vi "motioncontrol.vi"() -> ()   [LabVIEW 2016]
uses:
  GitHub/UCSB-Gantry/V5/Drivers/Aerotech A3200/Motion/MoveAbsSingle.vi
  GitHub/UCSB-Gantry/V5/Drivers/Aerotech A3200/Aerotech VIs.lvlib
panel:
  in  "Radius":dbl
  in  "Y Endpoint":dbl
  in  "X Endpoint":dbl
  in  "Make Circle":bool
  out "Z Position":dbl
  out "X Position":dbl
  out "Theta Position":dbl
  out "Y Position":dbl
  in  "Joystick ON/OFF":bool
  in  "Incrimental":bool
  in  "Angular position":dbl
  in  "Angular rotation":dbl
  in  "Theta-Go":bool
  in  "Abs distance":dbl
  in  "Incrimental":bool
  in  "Inc distance":dbl
  in  "Z-Go":bool
  in  "Square Speeds":dbl[](array[numeric])=[0.0, 0.0, 0.0]
  in  "Square Sizes":dbl[](array[numeric])=[0.0, 0.0, 0.0]
  in  "XY Go":bool
  in  "Make CW square":bool
  in  "positions/abs":dbl[](array[numeric])=[0.0, 0.0]
  in  "distances/linear":dbl[](array[numeric])=[0.0, 0.0]
  in  "Linear":bool
  in  "STOP PROGRAM":bool
  # "XY Motion"
  # "Theta"
  # "X"
  # "Y"
  # "Absolute"
  # "abs"
  # "Z-Control"
  # "Shapes"
  # "Absolute"
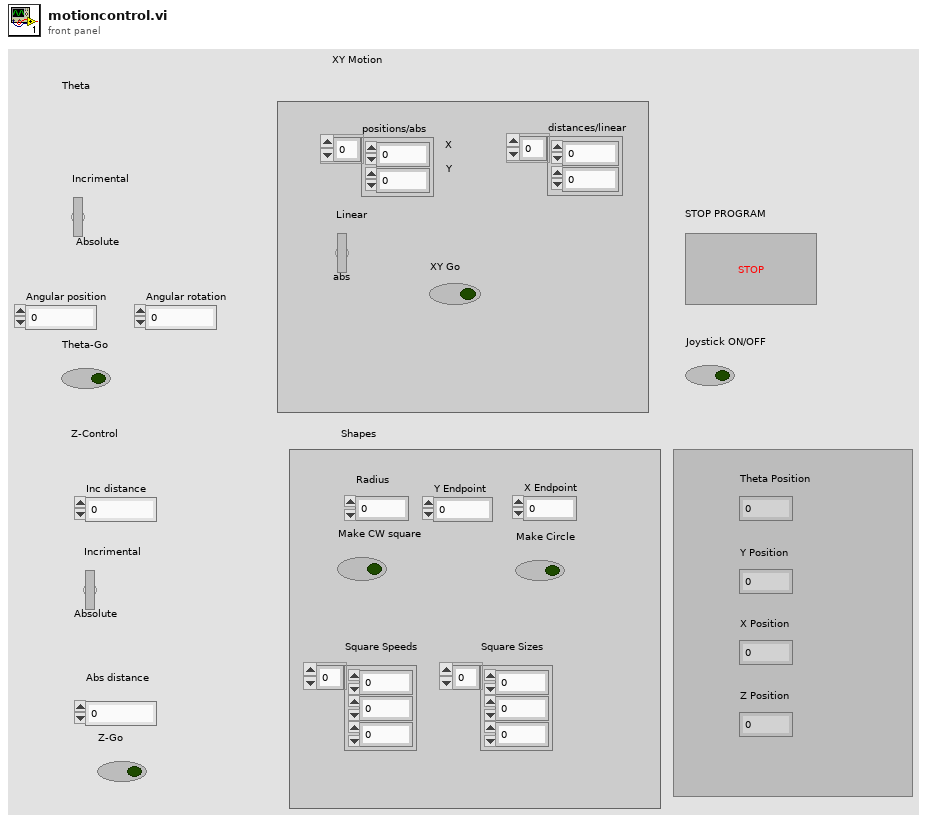
[diagram p1: front panel]
types:
  T1 = typedef "Aerotech VIs.lvlib/ControllerDiagPacket.ctl" = cluster{"Number of Diag Packets":i32, "Axes":T2[], "error":errorcluster}
  T2 = typedef "Aerotech VIs.lvlib/AxisDiagPacket.ctl" = cluster{"Axis Name":string, "Analog Input 0":dbl, "Analog Input 1":dbl, "Axis Fault (num)":i32, "Axis Fault (str)":string, "Axis Fault (bits)":cluster{"AmplifierFault":bool, "AmplifierTemperatureFault":bool, "CcwEndOfTravelLimitFault":bool, "CcwSoftwareLimitFault":bool, "CommunicationLostFault":bool, "CwEndOfTravelLimitFault":bool, "CwSoftwareLimitFault":bool, "EmergencyStopFault":bool, "EncoderFault":bool, "ExternalFault":bool, "FeedbackScalingFault":bool, "GantryMisalignFault ":bool, "HallSensorFault":bool, "InPositionTimeoutFault":bool, "MarkerSearchFault":bool, "MaxVelocityCommandFault":bool, "MotorTemperatureFault":bool, "None":bool, "OverCurrentFault":bool, "PositionErrorFault":bool, "PositionFeedbackFault":bool, "PowerSupplyFault":bool, "ProbeInputFault":bool, "SafeZoneFault":bool, "VelocityErrorFault":bool, "VelocityFeedbackFault":bool, "VoltageClampFault":bool}, "Axis Status (num)":i32, "Axis Status (str)":string, "Axis Status (bits)":cluster{"BacklashActive":bool, "CalibrationEnabled1D":bool, "CalibrationEnabled2D":bool, "CommandValid":bool, "DriveAbortPending":bool, "DrivePending":bool, "Enabling":bool, "GainMappingEnabled":bool, "GantryAligned":bool, "GantryRealigning":bool, "Homed":bool, "Homing":bool, "IFOVEnabled":bool, "JogGenerating":bool, "Jogging":bool, "JoystickControl":bool, "MasterSlaveControl":bool, "MotionBlocked":bool, "MotionClamped":bool, "MoveDone":bool, "None":bool, "NotVirtual":bool, "Profiling":bool, "Stability0":bool, "Stability1":bool, "TrajectoryFiltering":bool, "WaitDone":bool}, "Current Command":sgl, "Current Error":sgl, "Current Feedback":sgl, "Digital Inputs":i32, "Digital Outputs":i32, "Drive Status":i32, "Drive Status (str)":string, "Drive Status (bits)":cluster{"AccelerationPhase":bool, "AutofocusActive":bool, "BrakeOutput":bool, "CcwEndOfTravelLimitInput":bool, "CosineEncoderError":bool, "CurrentClamp":bool, "CwEndOfTravelLimitInput":bool, "DecelerationPhase":bool, "DualLoopActive":bool, "EmergencyStopInput":bool, "Enabled":bool, "EncoderClipping":bool, "GalvoCalibrationEnabled":bool, "GalvoPowerCorrection":bool, "HallAInput":bool, "HallBInput":bool, "HallCInput":bool, "HighResolutionMode":bool, "HomeLimitInput":bool, "InPosition":bool, "InPosition2":bool, "MarkerInput":bool, "MarkerLatch":bool, "MoveActive":bool, "NoMotorSupply":bool, "None":bool, "PowerLimiting":bool, "ProgrammingFlash":bool, "ProgrammingMXH":bool, "PSOHaltLatch":bool, "ServoControl":bool, "SineEncoderError":bool}, "Position Feedback Auxiliary":dbl, "Position Command":dbl, "Position Error":dbl, "Position Feedback":dbl, "Program Position Command":dbl, "Program Position Error":dbl, "Program Position Feedback":dbl, "Velocity Command":dbl, "Velocity Error":dbl, "Velocity Feedback":dbl}
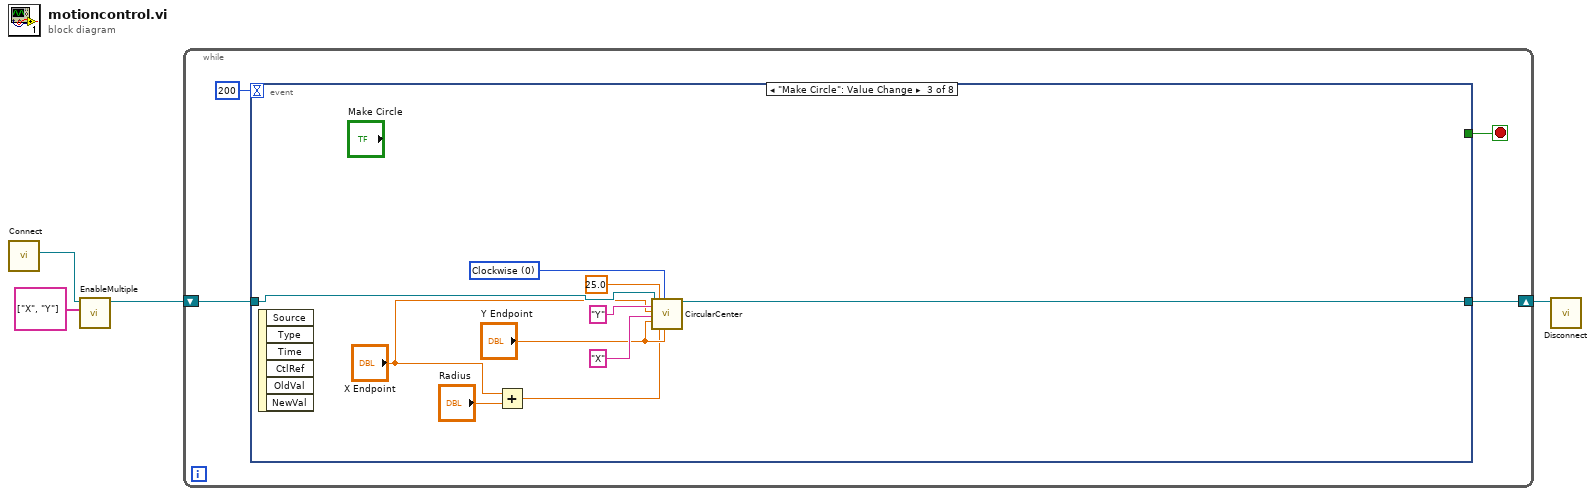
[diagram p0: block diagram]
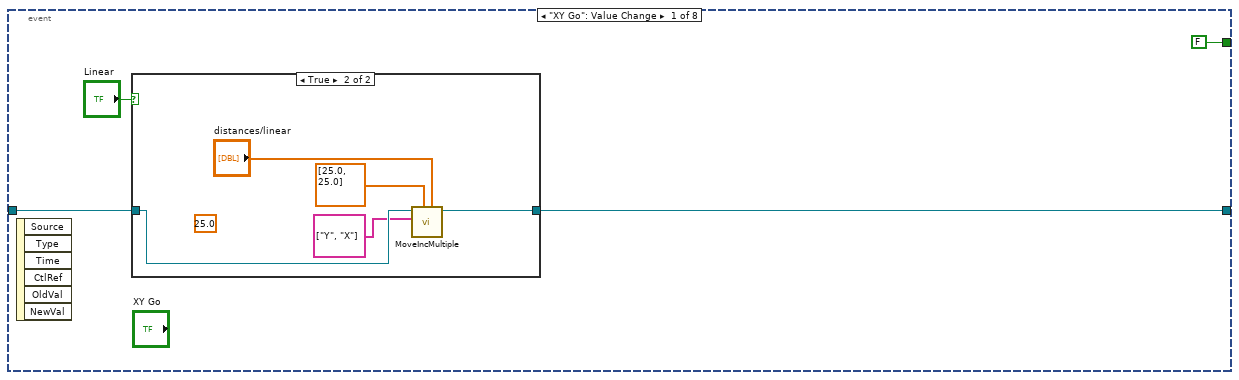
[diagram p2: hidden frame]
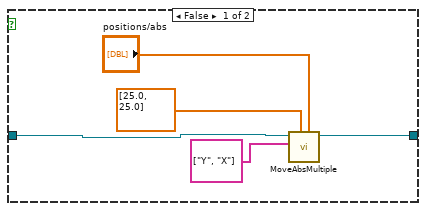
[diagram p3: hidden frame]
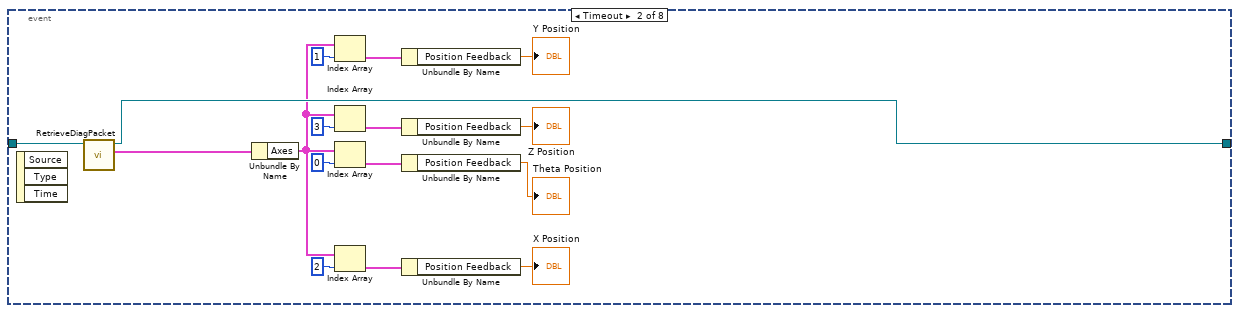
[diagram p4: hidden frame]
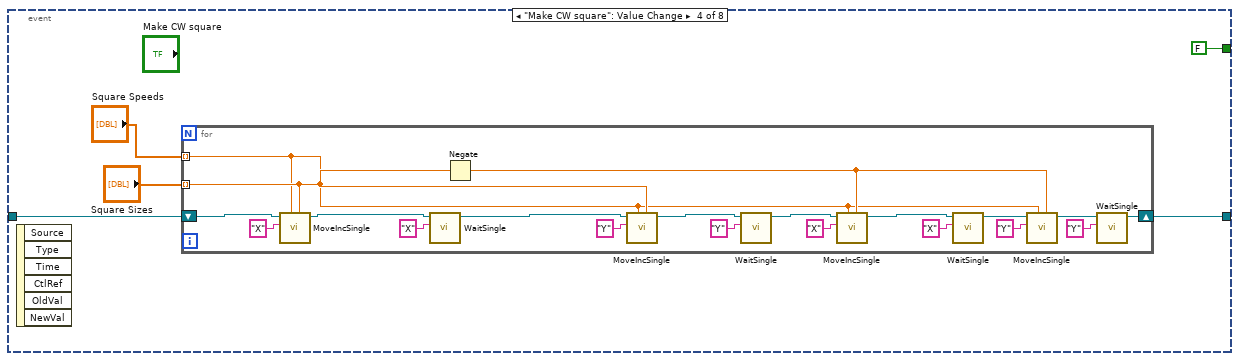
[diagram p5: hidden frame]
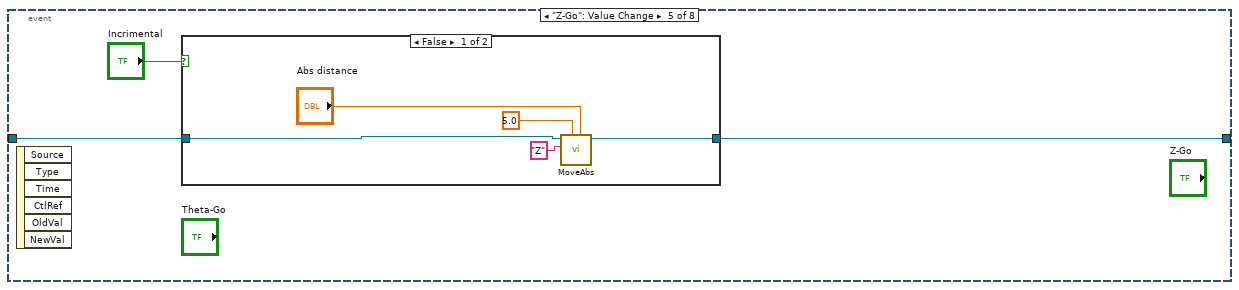
[diagram p6: hidden frame]
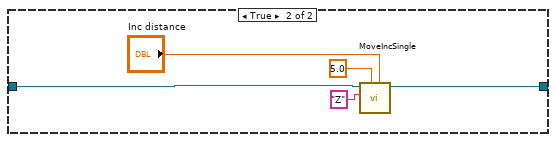
[diagram p7: hidden frame]
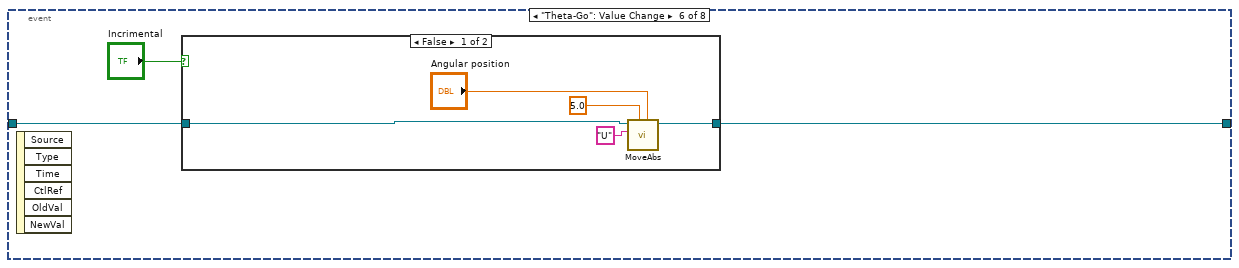
[diagram p8: hidden frame]
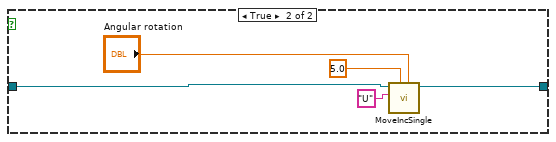
[diagram p9: hidden frame]
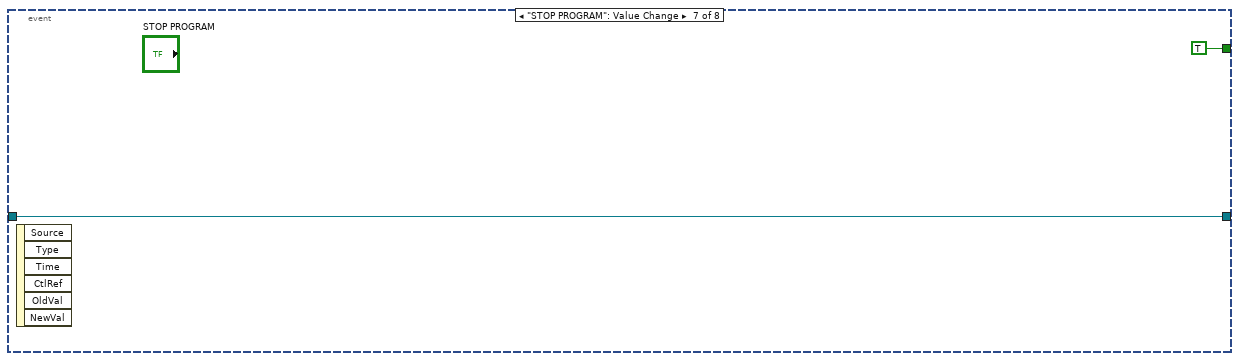
[diagram p10: hidden frame]
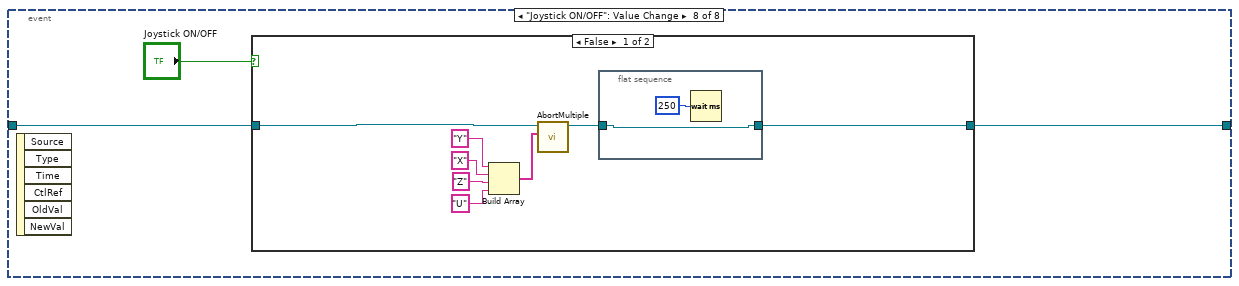
[diagram p11: hidden frame]
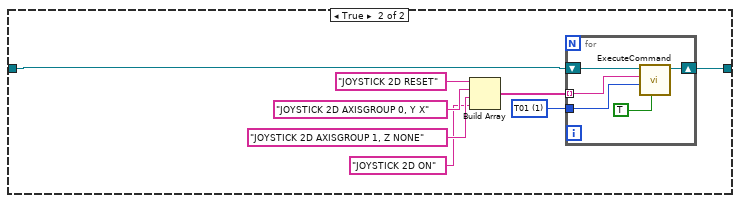
[diagram p12: hidden frame]
diagram:
  n1 = call "Connect.vi"() -> ("controller"=w4:refnum<k24>)  [unwired: 10 in, 1 out]
  n2 = call "EnableMultiple.vi"("axis names"=string[] ["X", "Y"], "controller in"=w4) -> ("controller out"=w2:refnum<k24>)  [unwired: 8 in, 1 out]
  n3 = while {
    shift-right: [w6] -> w1
    shift-left: w2 -> [w8]
    stop <- w7 stop-if-true
    n4 = event shown="[2] \"Make Circle\": Value Change" {
      selector: _ -> [_ _ _ _ _ _ _ _]
      dyn-events: _ -> [_ _ _ _ _ _ _ _]
      timeout: 200 -> [_ _ _ _ _ _ _ _]
      tunnel: w8 -> [w9 w38 w48 w49 w74 w87 w100 w104]
      tunnel: [FALSE _ _ FALSE _ _ TRUE _] -> w7
      tunnel: [w10 w36 w44 w53 w76 w88 w100 w103] -> w6
      event "XY Go": Value Change {
        n5 = event-data() -> ()  [unwired: 1 in, 6 out]
        n6 = case shown="True" "Linear" {
          tunnel: w9 -> [w17 w22]
          tunnel: [w13 w18] -> w10
          frame False {
            n7 = call "MoveAbsMultiple.vi"("positions"="positions/abs", "speeds"=dbl[] [25.0, 25.0], "axis names"=string[] ["Y", "X"], "controller in"=w17) -> ("controller out"=w13:refnum<k24>)  [unwired: 6 in, 1 out]
          }
          frame True {
            (unwired) 25.0 ("speed")
            n8 = call "MoveIncMultiple.vi"("distances"="distances/linear", "speeds"=dbl[] [25.0, 25.0], "axis names"=string[] ["Y", "X"], "controller in"=w22) -> ("controller out"=w18:refnum<k24>)  [unwired: 6 in, 1 out]
          }
        }
      }
      event Timeout {
        n9 = event-data() -> ()  [unwired: 1 in, 3 out]
        n10 = call "RetrieveDiagPacket.vi"("Controller In"=w38) -> ("ControllerDiagPacket"=w37:T1, "Controller Out"=w36:refnum<k24>)  [unwired: 8 in, 1 out]
        n11 = Unbundle By Name(w37) -> ("Axes"=w23:T2[])
        n12 = Index Array(array=w23, index=1) -> (element=w34:T2)
        n13 = Index Array(array=w23, index=3) -> (element=w28:T2)
        n14 = Index Array(array=w23, index=0) -> (element=w31:T2)
        n15 = Index Array(array=w23, index=2) -> (element=w29:T2)
        n16 = Unbundle By Name(w34) -> ("Position Feedback"=→"Y Position":dbl)
        n17 = Unbundle By Name(w28) -> ("Position Feedback"=→"Z Position":dbl)
        n18 = Unbundle By Name(w31) -> ("Position Feedback"=→"Theta Position":dbl)
        n19 = Unbundle By Name(w29) -> ("Position Feedback"=→"X Position":dbl)
      }
      event "Make Circle": Value Change {
        w43 = u16 0 items=["Clockwise", "Counter-clockwise"] ("direction")
        n20 = event-data() -> ()  [unwired: 1 in, 6 out]
        n21 = Add(x="X Endpoint", y="Radius") -> (x+y=w39:dbl)
        n22 = call "CircularCenter.vi"("controller in"=w48, "axis 1 name"="Y", "axis 1 endpoint"="X Endpoint", "axis 2 name"="X", "axis 2 endpoint"="Y Endpoint", "speed"=25.0, "axis 1 center point"=w39, "direction"=w43, "axis 2 center point"="Y Endpoint") -> ("controller out"=w44:refnum<k24>)  [unwired: 9 in, 1 out]
      }
      event "Make CW square": Value Change {
        n23 = event-data() -> ()  [unwired: 1 in, 6 out]
        n24 = for {
          shift-right: [w56] -> w53
          shift-left: w49 -> [w67]
          tunnel: "Square Sizes" -> [w72] mode=indexing
          tunnel: "Square Speeds" -> [w54] mode=indexing
          n25 = call "MoveIncSingle.vi"("distance"=w72, "speed"=w54, "axis name"="X", "controller in"=w67) -> ("controller out"=w66:refnum<k24>)  [unwired: 6 in, 1 out]
          n26 = call "WaitSingle.vi"("axis name"="X", "controller in"=w66) -> ("controller out"=w65:refnum<k24>)  [unwired: 7 in, 2 out]
          n27 = Negate(x=w72) -> (-x=w71:dbl)
          n28 = call "MoveIncSingle.vi"("distance"=w72, "speed"=w54, "axis name"="Y", "controller in"=w65) -> ("controller out"=w63:refnum<k24>)  [unwired: 6 in, 1 out]
          n29 = call "WaitSingle.vi"("axis name"="Y", "controller in"=w63) -> ("controller out"=w62:refnum<k24>)  [unwired: 7 in, 2 out]
          n30 = call "MoveIncSingle.vi"("distance"=w71, "speed"=w54, "axis name"="X", "controller in"=w62) -> ("controller out"=w60:refnum<k24>)  [unwired: 6 in, 1 out]
          n31 = call "WaitSingle.vi"("axis name"="X", "controller in"=w60) -> ("controller out"=w59:refnum<k24>)  [unwired: 7 in, 2 out]
          n32 = call "MoveIncSingle.vi"("distance"=w71, "speed"=w54, "axis name"="Y", "controller in"=w59) -> ("controller out"=w57:refnum<k24>)  [unwired: 6 in, 1 out]
          n33 = call "WaitSingle.vi"("axis name"="Y", "controller in"=w57) -> ("controller out"=w56:refnum<k24>)  [unwired: 7 in, 2 out]
        }
      }
      event "Z-Go": Value Change {
        n34 = event-data() -> ()  [unwired: 1 in, 6 out]
        n35 = case shown="False" "Incrimental" {
          tunnel: w74 -> [w78 w86]
          tunnel: [w77 w82] -> w76
          frame False {
            n36 = call-poly "MoveAbs.vi"("position"="Abs distance", "speed"=5.0, "axis name"="Z", "controller in"=w78) -> ("controller out"=w77:refnum<k24>)  [unwired: 6 in, 1 out]
          }
          frame True {
            n37 = call "MoveIncSingle.vi"("distance"="Inc distance", "speed"=5.0, "axis name"="Z", "controller in"=w86) -> ("controller out"=w82:refnum<k24>)  [unwired: 6 in, 1 out]
          }
        }
      }
      event "Theta-Go": Value Change {
        n38 = event-data() -> ()  [unwired: 1 in, 6 out]
        n39 = case shown="False" "Incrimental" {
          tunnel: w87 -> [w91 w96]
          tunnel: [w90 w95] -> w88
          frame False {
            n40 = call-poly "MoveAbs.vi"("position"="Angular position", "speed"=5.0, "axis name"="U", "controller in"=w91) -> ("controller out"=w90:refnum<k24>)  [unwired: 6 in, 1 out]
          }
          frame True {
            n41 = call "MoveIncSingle.vi"("distance"="Angular rotation", "speed"=5.0, "axis name"="U", "controller in"=w96) -> ("controller out"=w95:refnum<k24>)  [unwired: 6 in, 1 out]
          }
        }
      }
      event "STOP PROGRAM": Value Change {
        n42 = event-data() -> ()  [unwired: 1 in, 6 out]
      }
      event "Joystick ON/OFF": Value Change {
        n43 = event-data() -> ()  [unwired: 1 in, 6 out]
        n44 = case shown="False" "Joystick ON/OFF" {
          tunnel: w104 -> [w106 w116]
          tunnel: [w105 w115] -> w103
          frame False {
            n45 = Build Array("Y" ("axis name"), "X", "Z", "U") -> (w108:string[])
            n46 = call "AbortMultiple.vi"("axis names"=w108, "controller in"=w106) -> ("controller out"=w107:refnum<k24>)  [unwired: 8 in, 1 out]
            n47 = flat-sequence {
              tunnel: w107 -> [w114]
              tunnel: [w114] -> w105
              frame #0 {
                n48 = Wait (ms)(milliseconds to wait=u32 250) -> ()  [unwired: 1 out]
              }
            }
          }
          frame True {
            w118 = 1 items=["TLibrary", "T01", "T02", "T03", "T04", "T05", "T06", "T07", "T08", "T09", "T10", "T11", "T12", "T13", "T14", "T15", "T16", "T17", "T18", "T19", "T20", "T21", "T22", "T23", "T24", "T25", "T26", "T27", "T28", "T29", "T30", "T31"] ("taskId")
            n49 = Build Array("JOYSTICK 2D RESET", "JOYSTICK 2D AXISGROUP 0, Y X", "JOYSTICK 2D AXISGROUP 1, Z NONE", "JOYSTICK 2D ON") -> (w119:string[])
            n50 = for {
              tunnel: w119 -> [w127] mode=indexing
              tunnel: w118 -> [w126]
              shift-right: [w123] -> w115
              shift-left: w116 -> [w125]
              n51 = call "ExecuteCommand.vi"("return immediately"=TRUE, "taskId"=w126, "Command Code"=w127, "controller in"=w125) -> ("controller out"=w123:refnum<k24>)  [unwired: 5 in, 2 out]
            }
          }
        }
      }
    }
  }
  n52 = call "Disconnect.vi"("controller"=w1) -> ()  [unwired: 10 in, 1 out]
